vi "Set Plot Axis.vi"(9 "Waveform Array":waveform(dbl)[](array[waveform]), 10 "Large Scale threshhold":dbl=10.0 format="%#_13g", 11 "Waveform Chart ref":refnum<vi>) -> (1 "Waveform Array out":waveform(dbl)[](array[waveform]))   [LabVIEW 2021]
doc: "Move each plot to the Y Axis that matches its magnitude according to threshhold.\n\n- Small signals on axis 0\n- Large signals on axis 1"
panel:
  out "error out":errorcluster
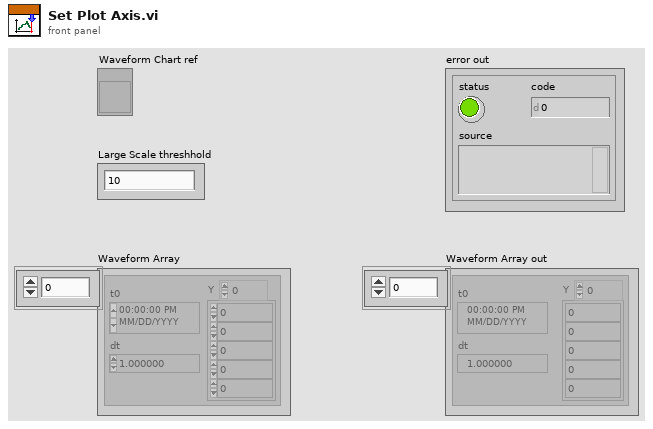
[diagram p1: front panel]
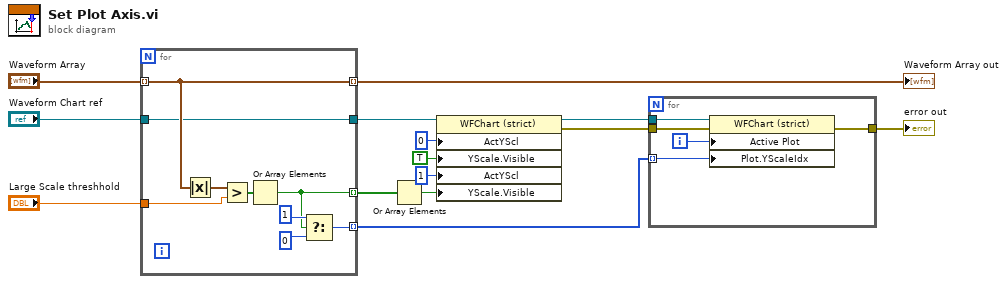
[diagram p0: block diagram]
diagram:
  n1 = for {
    tunnel: [w23] -> w14 mode=indexing
    tunnel: "Waveform Array" -> [w23] mode=indexing
    tunnel: "Waveform Chart ref" -> [w15]
    tunnel: [w18] -> w11 mode=indexing
    tunnel: [w15] -> w10
    tunnel: "Large Scale threshhold" -> [w17]
    tunnel: [w16] -> w2 mode=indexing
    n2 = Absolute Value(x=w23) -> (abs(x)=w19:waveform(dbl))
    n3 = Greater?(x=w19, y=w17) -> (0:w22:bool[])
    n4 = Or Array Elements(Boolean array=w22) -> (logical OR=w18:bool)
    n5 = Select(t=u32 1 ("Plot.Y Scale Index"), s=w18, f=u32 0 ("Plot.Y Scale Index")) -> (s? t:f=w16:u32)
  }
  "Waveform Array out" <- w14
  n6 = Or Array Elements(Boolean array=w11) -> (logical OR=w9:bool)
  n7 = property class="WFChart (strict)"(reference=w10, "ActYScl"=0 ("Active Y Scale"), "YScale.Visible"=TRUE ("Y Scale.Visible"), "ActYScl"=1 ("Active Y Scale"), "YScale.Visible"=w9) -> (reference out=w3:refnum<vi>, error out=w4:errorcluster)  [unwired: 1 in]
  n8 = for {
    tunnel: w4 -> [w28]
    tunnel: w3 -> [w27]
    tunnel: [w26] -> w1
    tunnel: w2 -> [w24] mode=indexing
    i -> [w25]
    n9 = property class="WFChart (strict)"(reference=w27, error in=w28, "Active Plot"=w25, "Plot.YScaleIdx"=w24) -> (error out=w26:errorcluster)  [unwired: 1 out]
  }
  "error out" <- w1
